vi "Select Device.vi"(4 "error in (no error)":errorcluster, 7 "Device":i32) -> (0 "error out":errorcluster, 2 "function return":i32)   [LabVIEW 2020, in "MPH16.lvlib"]
doc: "long SelectDevice(const long Device);"
uses:
  MPH16.lvlib
  ThorPinholeStepper.dll
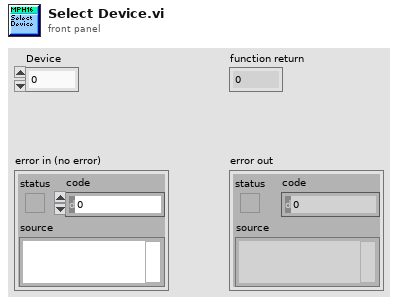
[diagram p1: front panel]
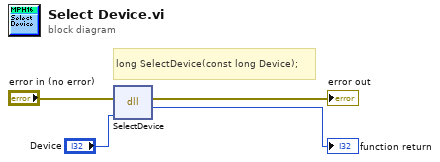
[diagram p0: block diagram]
diagram:
  # "long SelectDevice(const long Device);"
  n1 = dll-call lib="D:/software/TweezerTron Project/Instruments/Thorlabs/MPH_SDK/ThorPinholeStepper.dll" fn="SelectDevice"(error in="error in (no error)", "Device"="Device") -> (error out=→"error out":errorcluster, "return type"=→"function return":i32)  [unwired: 3 in, 1 out]
